vi "Fpga-AXI-Stream-Test.2.vi"() -> ()   [LabVIEW 2017]
uses:
  <vilib>/Platform/TimedLoop/XDataNode/XDataNode.xnode
  <vilib>/Platform/TimedLoop/XDataNode/nitl_modes.ctl
  <vilib>/Platform/TimedLoop/XDataNode/XDNodeRunTimeDep.lvlib
  <vilib>/Platform/TimedLoop/XDataNode/wakeup.ctl
  <vilib>/Platform/TimedLoop/XDataNode/timing_clust.ctl
  <vilib>/rvi/IPIntegrationNode/IPINode_Xnode/niFpgaIPINode.xnode
  IP_BlockSimFiles/xsim.dir/d_microblaze_wrapper_top/xsimkD73A4B5A6D7649FD9F60D89D81179CEC.dll
  <vilib>/rvi/IPIntegrationNode/IPINode_Typedef/niFpgaIPINodeSupportedFamilies.ctl
  <vilib>/rvi/IPIntegrationNode/IPINode_Utilities/niFpgaIPINodeSimCore.vi
  <vilib>/rvi/DataTransferAndStorage/Container/XNode/niFpgaContainer.xnode
  <vilib>/rvi/interface/RandomDataEmulation/nirviRandomDataFpgaReadWriteTemplate.vi
panel:
  in  "sys_reset":bool
  in  "AXI_STR_RXD_tvalid":bool
  in  "AXI_STR_RXD_tlast":bool
  in  "AXI_STR_RXD_tdata":u32
  in  "AXI_STR_TXD_tready":bool
  out "AXI_STR_RXD_tready":bool
  out "AXI_STR_TXD_tvalid":bool
  out "AXI_STR_TXD_tlast":bool
  out "GPIO2_tri_o":u32
  out "AXI_STR_TXD_tdata":u32
  in  "GPIO1_tri_i":u32
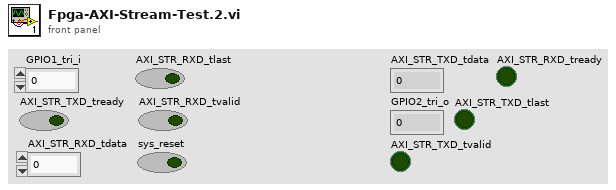
[diagram p1: front panel]
types:
  T1 = typedef "XDNodeRunTimeDep.lvlib/timing_clust.ctl" = cluster{"Expected End [f-1]":u64, "Actual End [f-1]":u64, "Finished Late? [f-1]":bool, "Expected End [i-1]":u64, "Actual End [i-1]":u64, "Finished Late? [i-1]":bool, "Expected Start [i]":u64, "Actual Start [i]":u64, "Expected Start [f]":u64, "Actual Start [f]":u64, "Source Name":string, "Structure Name":string, "Period":i64, "Deadline":i64, "Offset":i64, "Start":i64, "Priority":i32, "Timeout":i32, "Mode":T2, "Wakeup Reason":T3, "Error":errorcluster, "Source Type":string, "Secondary Source Type":string, "Global End Time":u64, "Global Start Time":u64, "Frame Duration":u64, "Iteration Duration":u64, "Assigned CPU":i32, "I/O Scan Engine Mode":u32}
  T2 = typedef "XDNodeRunTimeDep.lvlib/nitl_modes.ctl" = enum32{"No Change", "Process missed periods, maintain original phase", "Discard missed periods, maintain original phase", "Process missed periods, ignore original phase", "Discard missed periods, ignore original phase"}
  T3 = typedef "XDNodeRunTimeDep.lvlib/wakeup.ctl" = enum32{"Normal", "Aborted", "Asynchronous wakeup", "Timing source error", "Timed loop error", "Timeout"}
  T4 = typedef "niFpgaIPINodeSupportedFamilies.ctl" = cluster{"unlimited?":bool, "supported targets":string[]}
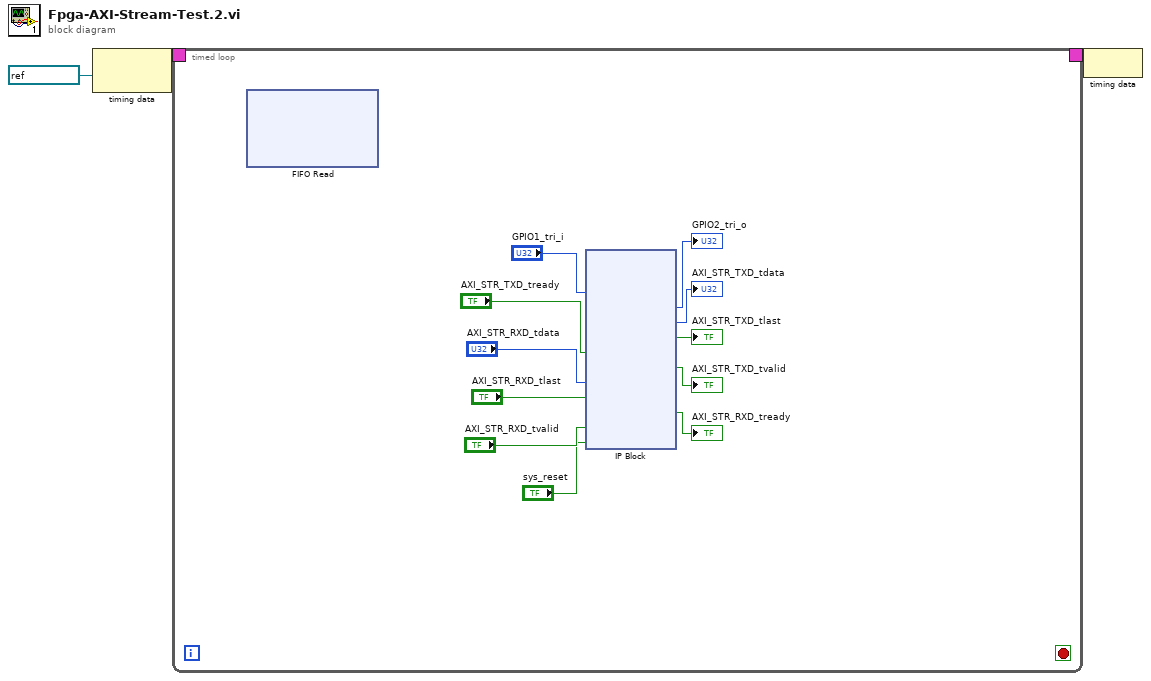
[diagram p0: block diagram]
diagram:
  n1 = node-c288(refnum<k21> "100MHz" ("Source Name")) -> (w3:T1)
  n2 = timed-loop {
    timing: w3 -> [_]
    timing-out: [_] -> w2
    stop <- _ stop-if-true
    n3 = xnode "FIFO Read"() -> ()  [unwired: 2 in, 3 out]
    n4 = xnode ("IP Block")("GPIO1_tri_i"="GPIO1_tri_i", "AXI_STR_TXD_tready"="AXI_STR_TXD_tready", "AXI_STR_RXD_tdata"="AXI_STR_RXD_tdata", "AXI_STR_RXD_tlast"="AXI_STR_RXD_tlast", "AXI_STR_RXD_tvalid"="AXI_STR_RXD_tvalid", "sys_reset"="sys_reset") -> ("GPIO2_tri_o"=→"GPIO2_tri_o":u32, "AXI_STR_TXD_tdata"=→"AXI_STR_TXD_tdata":u32, "AXI_STR_TXD_tlast"=→"AXI_STR_TXD_tlast":bool, "AXI_STR_TXD_tvalid"=→"AXI_STR_TXD_tvalid":bool, "AXI_STR_RXD_tready"=→"AXI_STR_RXD_tready":bool)  [unwired: 1 out]
  }
  n5 = node-c288(w2) -> ()
